vi "Initialise.vi"(4 "Default Timeout (ms)":i32=-1, 5 "Poll Interval (ms)":i32=10, 6 "Tag Root":string=".EVT", 7 "Event_Source.lvclass":refnum<class "Event_Source.lvclass">, 8 "error in (no error)":errorcluster, 9 "Tags to Create Events For":string[](array[string]), 10 "Buses":refnum<class "Bus_Access.lvclass">[](array[class]), 11 "Event_Bus in":refnum<class "Event_Bus.lvclass">) -> (0 "error out":errorcluster, 3 "Event_Bus out":refnum<class "Event_Bus.lvclass">)   [LabVIEW 2021, in "Event_Bus.lvclass"]
uses:
  Event_Bus.lvclass
  C:/TSA/Omni-Bus/Source/Omni-Bus/Bus Access/Bus_Access.lvclass
  Omni-Bus/Bus Access/Bus_Access.lvclass
  Support/Event Source/Polled_EventSource/Polled_EventSource.lvclass/Polled_EventSource.ctl
  Event_Bus.lvclass/Event_Bus.ctl
  Omni-Bus/Bus Access/Bus_Access.lvclass/Bus_Access.ctl
  Support/Event Source/Polled_EventSource/Properties/Write Poll Interval (ms).vi
  Properties/Write Buses.vi
  Properties/Write Tags to Event.vi
  Properties/Write Event_Source.vi
  Omni-Bus/Bus Access/Properties/Write Tag Root.vi
  Properties/Write Default Timeout (ms).vi
  Support/Event Source/Polled_EventSource/Polled_EventSource.lvclass
  C:/TSA/Omni-Bus/Source/Event Bus/Support/Event Source/Event_Source.lvclass
  C:/Program Files (x86)/National Instruments/LabVIEW 2021/vi.lib/TSA/Abstract Data Classes/Abs_Types/Type/Abs_Type.lvclass
  C:/TSA/Omni-Bus/Source/Event Bus/Support/Event Source/Polled_EventSource/Polled_EventSource.lvclass
  Support/Event Source/Event_Source.lvclass
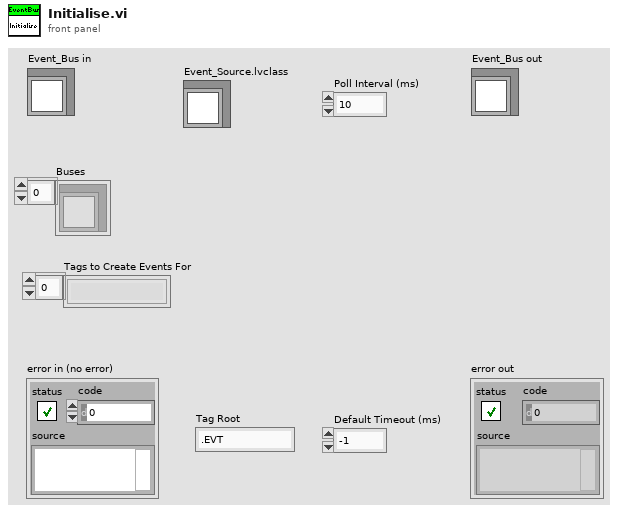
[diagram p1: front panel]
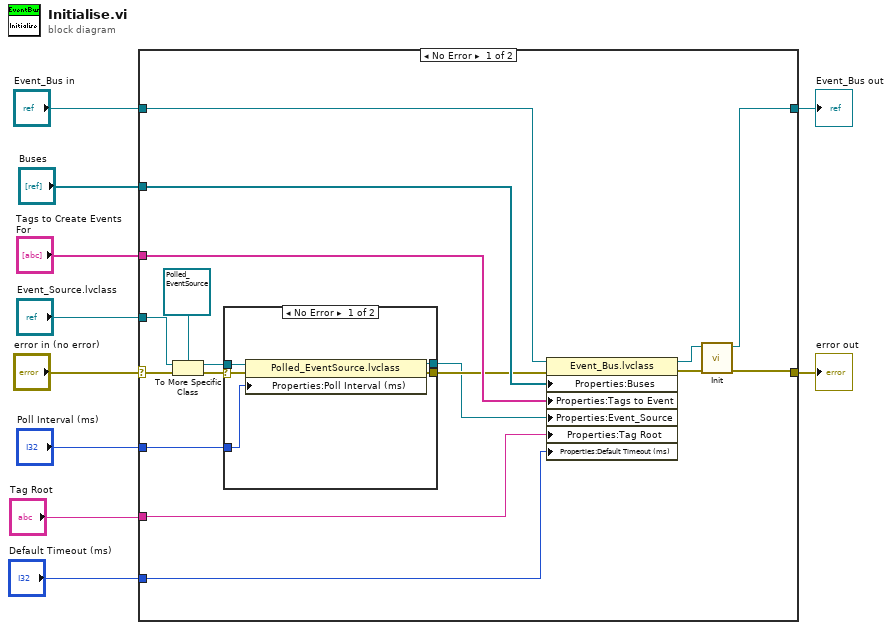
[diagram p0: block diagram]
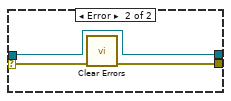
[diagram p2: hidden frame]
diagram:
  n1 = case shown="No Error" "error in (no error)" {
    selector: "error in (no error)" -> [w15 w37]
    tunnel: [w22 w37] -> w9
    tunnel: [w21 w36] -> w7
    tunnel: "Event_Bus in" -> [w27 w36]
    tunnel: "Buses" -> [w26 _]
    tunnel: "Tags to Create Events For" -> [w25 _]
    tunnel: "Tag Root" -> [w20 _]
    tunnel: "Default Timeout (ms)" -> [w19 _]
    tunnel: "Poll Interval (ms)" -> [w16 _]
    tunnel: "Event_Source.lvclass" -> [w13 _]
    frame No Error {
      n2 = To More Specific Class(target class=refnum<class "Polled_EventSource.lvclass"> refnum ("Polled_EventSource.lvclass"), reference=w13, error in=w15) -> (specific class reference=w11:refnum<class "Polled_EventSource.lvclass">, error out=w14:errorcluster)
      n3 = case shown="No Error" w14 {
        selector: w14 -> [w29 w35]
        tunnel: [w32 w34] -> w18
        tunnel: [w31 w33] -> w17
        tunnel: w16 -> [w30 _]
        tunnel: w11 -> [w28 w33]
        frame No Error {
          n4 = property class="Polled_EventSource.lvclass"(reference=w28, error in=w29, "Properties:Poll Interval (ms)"=w30) -> (reference out=w31:refnum<class "Polled_EventSource.lvclass">, error out=w32:errorcluster)
        }
        frame Error {
          n5 = call <vilib>:"Clear Errors.vi"("error in (no error)"=w35) -> ("error out"=w34:errorcluster)  [unwired: 5 in, 1 out]
        }
      }
      n6 = property class="Event_Bus.lvclass"(reference=w27, error in=w18, "Properties:Buses"=w26, "Properties:Tags to Event"=w25, "Properties:Event_Source"=w17, "Properties:Tag Root"=w20, "Properties:Default Timeout (ms)"=w19) -> (reference out=w23:refnum<class "Event_Bus.lvclass">, error out=w24:errorcluster)
      n7 = call-dynamic "Init.vi"("error in (no error)"=w24, "Data in"=w23) -> ("error out"=w22:errorcluster, "Data out"=w21:refnum<class "Event_Bus.lvclass">)  [unwired: 8 in]
    }
    frame Error {
    }
  }
  "error out" <- w9
  "Event_Bus out" <- w7
